vi "Unpack DRAM Word to LLP Packet.vi"(0 "dram word":T1, 1 "reset":bool, 2 "end of stream":bool, 5 "expected packet words":u64, 7 "packet word size":u16, 9 "input valid":bool, 12 "ready for output":bool=TRUE) -> (4 "tagged llp packet":T2, 6 "end of data":bool, 10 "output valid":bool, 14 "ready for input":bool)   [LabVIEW 2020, in "GettingStarted_Common_148X_FPGA.lvlib"]
uses:
  GettingStarted_Common_148X_FPGA.lvlib
  <instrlib>/FlexRIO/CSI-2/v2/FPGA/Types/Tagged LLP Packet.ctl
  <instrlib>/FlexRIO/CSI-2/v2/FPGA/Types/FPGA LLP Packet Tag.ctl
  <instrlib>/FlexRIO/CSI-2/v2/FPGA/Types/FPGA LLP Packet Timestamp.ctl
  <instrlib>/FlexRIO/CSI-2/v2/FPGA/Types/Timestamp ID.ctl
  <instrlib>/FlexRIO/CSI-2/v2/FPGA/Types/FPGA LLP Packet Size.ctl
  <instrlib>/FlexRIO/CSI-2/v2/FPGA/Types/LLP Packet.ctl
  <instrlib>/FlexRIO/CSI-2/v2/FPGA/Types/LLP Packet Header.ctl
  <instrlib>/FlexRIO/CSI-2/v2/FPGA/Types/LLP Packet Payload.ctl
  <instrlib>/FlexRIO/CSI-2/v2/FPGA/Types/LLP Packet Footer.ctl
  <instrlib>/_niInstr/Memory/v1/FPGA/Memory/Public/U256.ctl
  <instrlib>/_niInstr/Data Formatting/v1/FPGA/Private/Unpack/Unpack Impl.vi
  <instrlib>/_niInstr/Data Formatting/v1/FPGA/Private/Convert/Boolean Array to U8 Array.vi
  <instrlib>/_niInstr/Basic Elements/v1/FPGA/niInstr Basic Elements v1 FPGA.lvlib
  <instrlib>/_niInstr/Data Formatting/v1/FPGA/niInstr Data Formatting v1 FPGA.lvlib
  <instrlib>/_niInstr/Memory/v1/FPGA/Memory/niInstr Memory v1 FPGA.lvclass
  <instrlib>/FlexRIO/CSI-2/v2/FPGA/NI CSI-2 API FPGA v2.lvlib
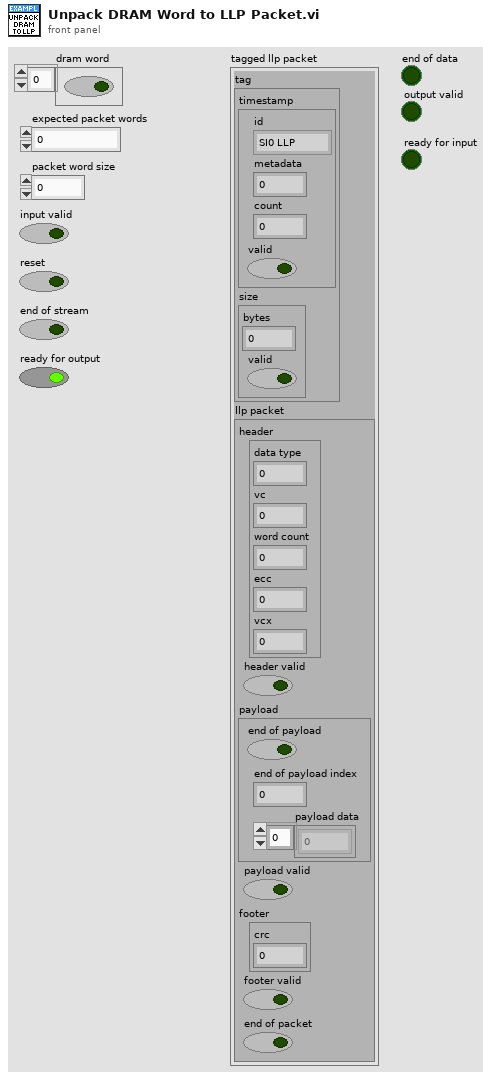
[diagram p1: front panel]
types:
  T1 = typedef "niInstr Memory v1 FPGA.lvclass/U256.ctl" = bool[]
  T2 = typedef "NI CSI-2 API FPGA v2.lvlib/Tagged LLP Packet.ctl" = cluster{"tag":T3, "llp packet":T7}
  T3 = typedef "NI CSI-2 API FPGA v2.lvlib/FPGA LLP Packet Tag.ctl" = cluster{"timestamp":T4, "size":T6}
  T4 = typedef "NI CSI-2 API FPGA v2.lvlib/FPGA LLP Packet Timestamp.ctl" = cluster{"valid":bool, "count":fxp<+,50,50>, "id":T5, "metadata":u8}
  T5 = typedef "NI CSI-2 API FPGA v2.lvlib/Timestamp ID.ctl" = enum8{"SI0 LLP", "SI1 LLP", "SI2 LLP", "SI3 LLP", "SI4 LLP", "SI5 LLP", "SI6 LLP", "SI7 LLP", "SO0 LLP", "SO1 LLP", "SO2 LLP", "SO3 LLP", "SO4 LLP", "SO5 LLP", "SO6 LLP", "SO7 LLP", "Ser0 GPIO Bank", "Ser1 GPIO Bank", "Ser2 GPIO Bank", "Ser3 GPIO Bank", "Ser4 GPIO Bank", "Ser5 GPIO Bank", "Ser6 GPIO Bank", "Ser7 GPIO Bank", "Des0 GPIO Bank", "Des1 GPIO Bank", "Des2 GPIO Bank", "Des3 GPIO Bank", "Des4 GPIO Bank", "Des5 GPIO Bank", "Des6 GPIO Bank", "Des7 GPIO Bank", "User0", "User1", "User2", "User3", "User4", "User5", "User6", "User7", "User8", "User9", "User10", "User11", "User12", "User13", "User14", "User15", "User16", "User17", "User18", "User19", "User20", "User21", "User22", "User23", "User24", "User25", "User26", "User27", "User28", "User29", "User30", "User31"}
  T6 = typedef "NI CSI-2 API FPGA v2.lvlib/FPGA LLP Packet Size.ctl" = cluster{"bytes":fxp<+,17,17>, "valid":bool}
  T7 = typedef "NI CSI-2 API FPGA v2.lvlib/LLP Packet.ctl" = cluster{"header":T8, "header valid":bool, "payload":T9, "payload valid":bool, "footer":T10, "footer valid":bool, "end of packet":bool}
  T8 = typedef "NI CSI-2 API FPGA v2.lvlib/LLP Packet Header.ctl" = cluster{"word count":u16, "ecc":fxp<+,6,6>, "vcx":fxp<+,2,2>, "data type":fxp<+,6,6>, "vc":fxp<+,2,2>}
  T9 = typedef "NI CSI-2 API FPGA v2.lvlib/LLP Packet Payload.ctl" = cluster{"end of payload":bool, "end of payload index":fxp<+,3,3>, "payload data":u8[]}
  T10 = typedef "NI CSI-2 API FPGA v2.lvlib/LLP Packet Footer.ctl" = cluster{"crc":u16}
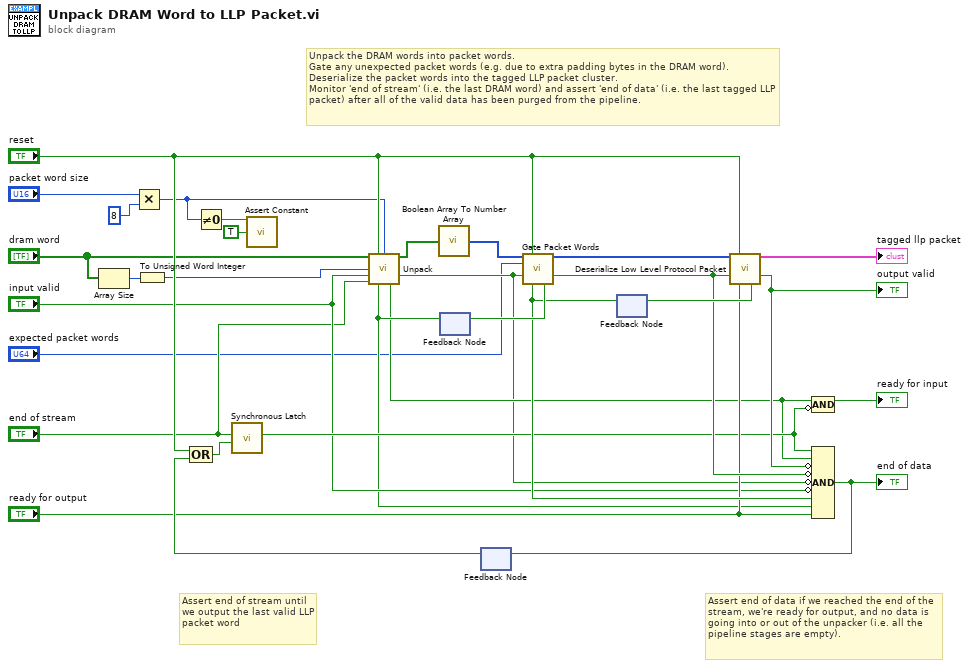
[diagram p0: block diagram]
diagram:
  # "Unpack the DRAM words into packet words.\nGate any unexpected packet words (e.g. due to extra padding bytes in the DRAM word).\nDeserialize the packet words into the tagged LLP packet cluster.\nMonitor 'end of stream' (i.e. the last DRAM word) and assert 'end of data' (i.e. the last tagged LLP packet) after all of the valid data has been purged from the pipeline."
  # "Assert end of data if we reached the end of the stream, we're ready for output, and no data is going into or out of the unpacker (i.e. all the pipeline stages are empty)."
  # "Assert end of stream until we output the last valid LLP packet word"
  n1 = Array Size(array="dram word") -> (size(s)=w15:i32)
  n2 = Multiply(x="packet word size", y=u16 8) -> (x*y=w4:u16)
  n3 = To Unsigned Word Integer(number=w15) -> (unsigned 16bit integer=w14:u16)
  n4 = Not Equal To 0?(x=w4) -> (x != 0?=w6:bool)
  n5 = call <instrlib>:"Assert Constant.vi"("constant terminal"=w6, "enable show error"=TRUE) -> ()  [unwired: 14 in]
  n6 = feedback #1() -> (w13:bool)  [unwired: 1 in]
  n7 = call-poly <instrlib>:"Unpack.vi"("data in"="dram word", "reset"="reset", "output data size (bits)"=w4, "valid data size (bits)"=w14, "input valid"="input valid", "end of stream"="end of stream", "ready for output"=w13) -> ("data out"=w9:bool[], "output valid"=w10:bool, "ready for input"=w12:bool)  [unwired: 6 in]
  n8 = call-poly <instrlib>:"Boolean Array To Number Array.vi"("data in"=w9) -> ("data out"=w1:u8[])  [unwired: 14 in]
  n9 = feedback #2() -> (w25:bool)  [unwired: 1 in]
  n10 = Compound Arithmetic op=OR("reset", w25) -> (w26:bool)
  n11 = call <instrlib>:"Synchronous Latch.vi"("clear"=w26, "set"="end of stream") -> ("out"=w18:bool)  [unwired: 9 in]
  n12 = feedback #3() -> (w20:bool)  [unwired: 1 in]
  n13 = call "Gate Packet Words.vi"("packet word in"=w1, "reset"="reset", "expected packet words"="expected packet words", "input valid"=w10, "ready for output"=w20) -> ("packet word out"=w27:u8[], "output valid out"=w21:bool, "ready for input"=w28:bool)  [unwired: 8 in]
  n14 = feedback-in #1(w28) -> ()
  n15 = call "Deserialize Low Level Protocol Packet.vi"("llp packet word"=w27, "reset"="reset", "input valid"=w21, "ready for output"="ready for output") -> ("tagged llp packet"=→"tagged llp packet":T2, "output valid"=w22:bool, "ready for input"=w29:bool)  [unwired: 9 in]
  "output valid" <- w22
  n16 = feedback-in #3(w29) -> ()
  n17 = Compound Arithmetic op=AND(w12, invert w18) -> (→"ready for input":bool)
  n18 = Compound Arithmetic op=AND(w18, w12, invert w22, invert w21, invert w10, invert "input valid", w20, w13, "ready for output") -> (w23:bool)
  "end of data" <- w23
  n19 = feedback-in #2(w23) -> ()
